vi "Decoder.vi"(8 "Joystick Data":string, 9 "Button Data":string, 10 "Conf":T3) -> (1 "Controller 2 State":T1={"Left X"=0, "Left Y"=0, "Right X"=0, "Right Y"=0, "Button Encoding 9-12"=0, "Button Encoding 1-8"=0, "POV"=-1} {"POV" items=["None"=-1, "POV Up"=0, "POV Up Right"=1, "POV Right"=2, "POV Down Right"=3, "POV Down"=4, "POV Down Left"=5, "POV Left"=6, "POV Up Left"=7]}, 2 "Controller 1 State":T1={"Left X"=0, "Left Y"=0, "Right X"=0, "Right Y"=0, "Button Encoding 9-12"=0, "Button Encoding 1-8"=0, "POV"=-1} {"POV" items=["None"=-1, "POV Up"=0, "POV Up Right"=1, "POV Right"=2, "POV Down Right"=3, "POV Down"=4, "POV Down Left"=5, "POV Left"=6, "POV Up Left"=7]})   [LabVIEW 2010, in "Packet Recorder.lvlib"]
uses:
  Packet Recorder.lvlib
  <vilib>/FTC/FTC ControllerState.ctl
  <vilib>/FTC/FTC POVState.ctl
  Components/Components.llb/Integer to Boolean Array_U32.vi
  Components/Components.lvlib
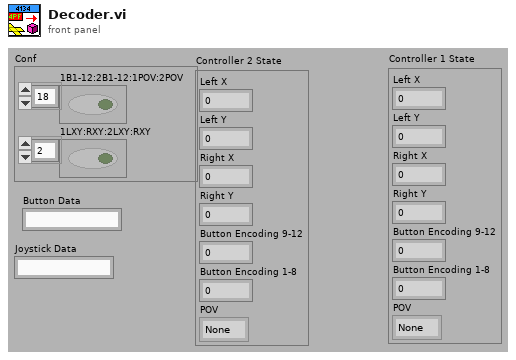
[diagram p1: front panel]
types:
  T1 = typedef "FTC ControllerState.ctl" = cluster{"Left X":i8, "Left Y":i8, "Right X":i8, "Right Y":i8, "Button Encoding 9-12":u8, "Button Encoding 1-8":u8, "POV":T2}
  T2 = typedef "FTC POVState.ctl" = i8
  T3 = cluster{"1B1-12:2B1-12:1POV:2POV":bool[], "1LXY:RXY:2LXY:RXY":bool[]}
  T4 = enum16{"big-endian, network order", "native, host order", "little-endian"}
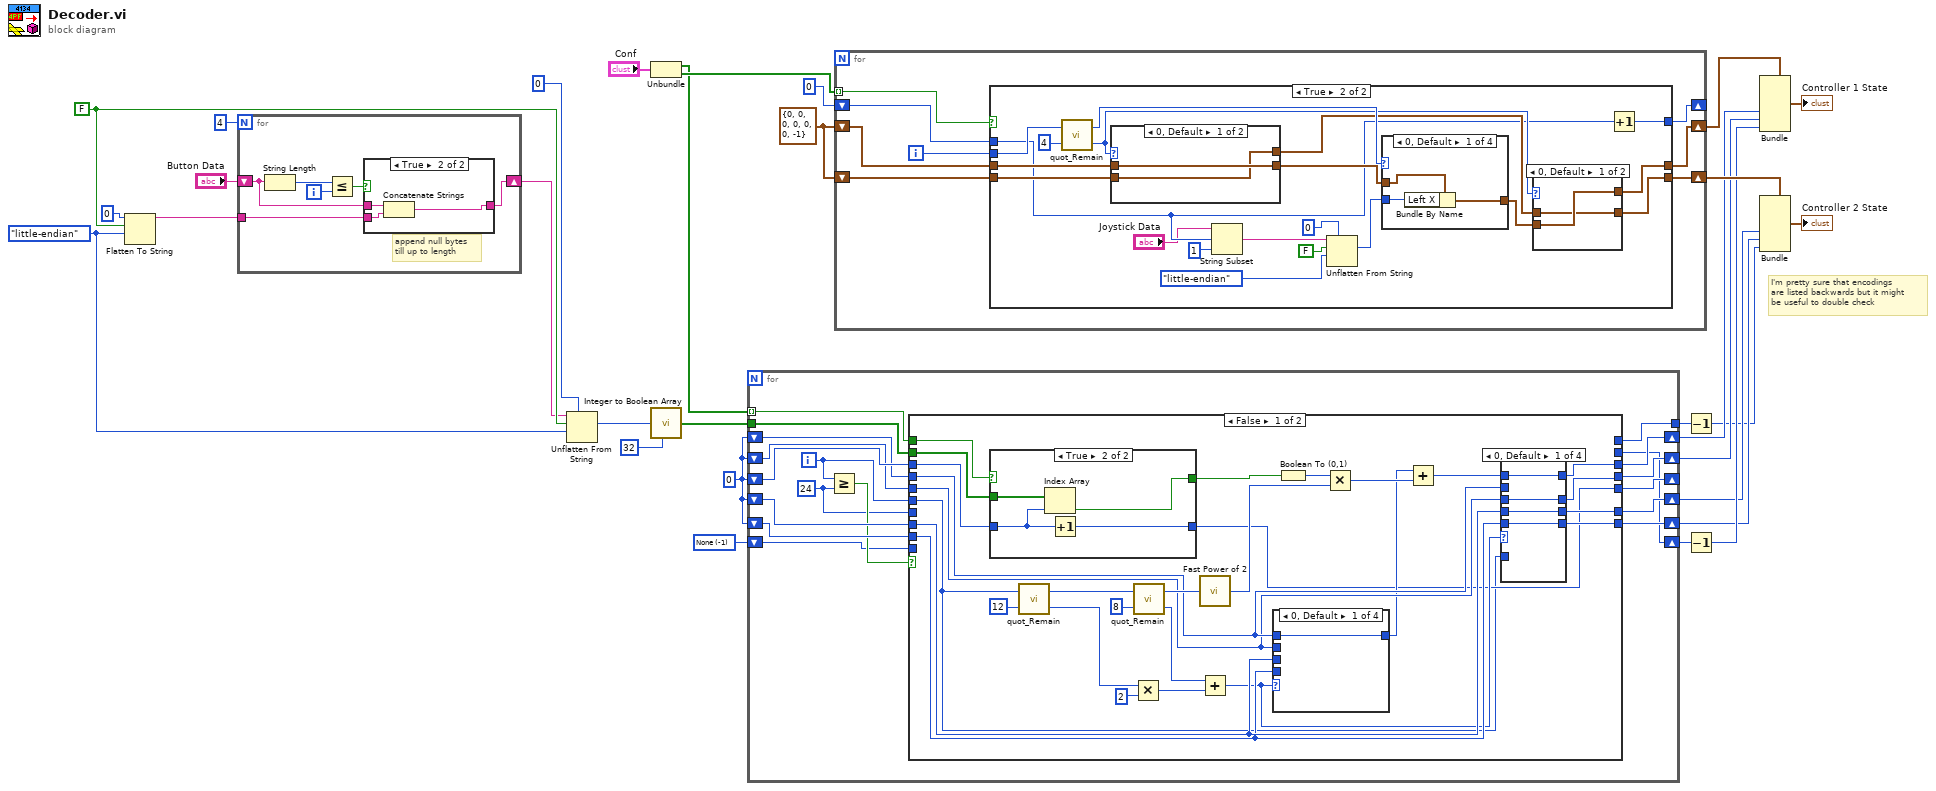
[diagram p0: block diagram]
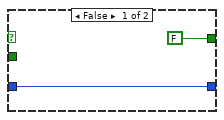
[diagram p9: hidden frame]
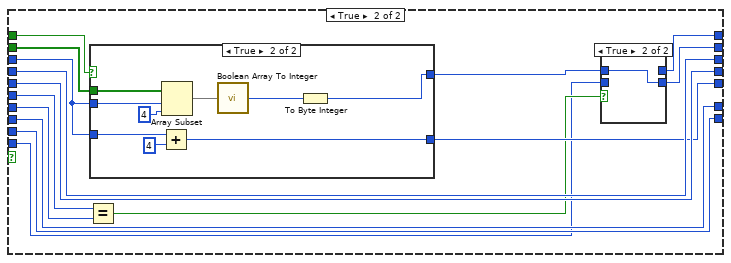
[diagram p10: hidden frame]
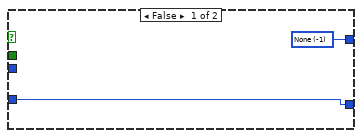
[diagram p12: hidden frame]
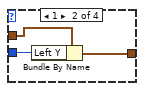
[diagram p16: hidden frame]
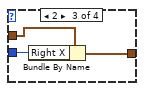
[diagram p17: hidden frame]
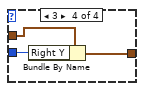
[diagram p18: hidden frame]
diagram:
  w11 = T2 -1 items=["None"=-1, "POV Up"=0, "POV Up Right"=1, "POV Right"=2, "POV Down Right"=3, "POV Down"=4, "POV Down Left"=5, "POV Left"=6, "POV Up Left"=7] ("POV")
  w17 = u8 0 ("index")
  w15 = FALSE ("data includes array or string size? (T)")
  w14 = T4."little-endian" ("byte order (0:big-endian, network order)")
  w28 = T1 {"Left X"=0, "Left Y"=0, "Right X"=0, "Right Y"=0, "Button Encoding 9-12"=0, "Button Encoding 1-8"=0, "POV"=-1} ("Controller 2 State")
  # "I'm pretty sure that encodings \nare listed backwards but it might\nbe useful to double check"
  n1 = Flatten To String(anything=u8 0, prepend array or string size? (T)=w15, byte order (0:big-endian, network order)=w14) -> (data string=w6:string)  [unwired: 1 in, 2 out]
  n2 = for {
    N: 4 -> [_]
    tunnel: w6 -> [w36]
    shift-right: [w35] -> w5
    shift-left: "Button Data" -> [w33]
    i -> [w32]
    # "append null bytes\ntill up to length"
    n3 = String Length(string=w33) -> (length=w34:i32)
    n4 = Less Or Equal?(x=w34, y=w32) -> (x <= y?=w31:bool)
    n5 = case shown="True" w31 {
      tunnel: w33 -> [w37 w40]
      tunnel: w36 -> [_ w39]
      tunnel: [w37 w38] -> w35
      frame False {
      }
      frame True {
        n6 = Concatenate Strings(w40, w39) -> (w38:string)
      }
    }
  }
  n7 = Unflatten From String(type=u32 0, binary string=w5, data includes array or string size? (T)=w15, byte order (0:big-endian, network order)=w14) -> (value=w9:u32)  [unwired: 1 in, 2 out]
  n8 = Unbundle("Conf") -> ("1B1-12:2B1-12:1POV:2POV"=w26:bool[], "1LXY:RXY:2LXY:RXY"=w27:bool[])
  n9 = call-poly "Integer to Boolean Array.vi"("number"=w9, "minimum"=u32 32) -> ("Boolean array"=w4:bool[])  [unwired: 5 in]
  n10 = for {
    tunnel: w26 -> [w58] mode=indexing
    tunnel: w4 -> [w57]
    shift-right: [w55] -> _
    shift-left: w17 -> [w56]
    shift-right: [w54] -> w19
    shift-left: w17 -> [w50]
    shift-right: [w51] -> w2
    shift-left: w17 -> [w47]
    shift-right: [w52] -> w3
    shift-left: w17 -> [w48]
    shift-right: [w53] -> w18
    shift-left: w17 -> [w49]
    shift-right: [w43] -> w13
    shift-left: w11 -> [w42]
    tunnel: [w41] -> w12
    i -> [w45]
    w44 = 24 ("y")
    n11 = Greater Or Equal?(x=w45, y=w44) -> (x >= y?=w46:bool)
    n12 = case shown="False" w46 {
      tunnel: w58 -> [w60 w121]
      tunnel: w57 -> [w86 w120]
      tunnel: w56 -> [w85 w119]
      tunnel: [w62 w123] -> w55
      tunnel: w45 -> [w59 w113]
      tunnel: [w73 w127] -> w54
      tunnel: [w72 w126] -> w53
      tunnel: [w71 w124] -> w52
      tunnel: [w70 w125] -> w51
      tunnel: w50 -> [w69 w127]
      tunnel: w49 -> [w68 w126]
      tunnel: w48 -> [w67 w124]
      tunnel: w47 -> [w66 w125]
      tunnel: w44 -> [_ w122]
      tunnel: [_ w116] -> w43
      tunnel: w42 -> [_ w115]
      tunnel: [_ w114] -> w41
      frame False {
        n13 = case shown="True" w60 {
          tunnel: w86 -> [_ w112]
          tunnel: w85 -> [w108 w111]
          tunnel: [w108 w110] -> w62
          tunnel: [FALSE w109] -> w61
          frame False {
          }
          frame True {
            n14 = Index Array(array=w112, index=w111) -> (element=w109:bool)
            n15 = Increment(x=w111) -> (x+1=w110:u8)
          }
        }
        n16 = call <vilib>:"quot_Remain.vi"("y"=12, "x"=w59) -> ("floor(x/y)"=w78:i32, "x-y*floor(x/y)"=w83:i32)
        n17 = Multiply(x=w78, y=2) -> (x*y=w76:i32)
        n18 = call <vilib>:"quot_Remain.vi"("y"=8, "x"=w83) -> ("floor(x/y)"=w75:i32, "x-y*floor(x/y)"=w81:i32)
        n19 = call "Fast Power of 2.vi"("power"=w81) -> ("result"=w80:u32)
        n20 = Add(x=w75, y=w76) -> (x+y=w63:i32)
        n21 = case shown="0, Default" w63 {
          tunnel: w69 -> [w87 _ _ _]
          tunnel: w68 -> [_ w88 _ _]
          tunnel: w67 -> [_ _ w89 _]
          tunnel: w66 -> [_ _ _ w90]
          tunnel: [w87 w88 w89 w90] -> w65
          frame 0, Default {
          }
          frame 1 {
          }
          frame 2 {
          }
          frame 3 {
          }
        }
        n22 = Boolean To (0,1)(Boolean=w61) -> (0, 1=w64:i16)
        n23 = Multiply(x=w64, y=w80) -> (x*y=w79:u32)
        n24 = Add(x=w65, y=w79) -> (x+y=w74:u32)
        n25 = case shown="0, Default" w63 {
          tunnel: w74 -> [w91 w98 w102 w106]
          tunnel: [w91 w97 w101 w105] -> w73
          tunnel: [w92 w98 w100 w104] -> w72
          tunnel: [w93 w96 w102 w103] -> w71
          tunnel: [w94 w95 w99 w106] -> w70
          tunnel: w66 -> [w94 w95 w99 _]
          tunnel: w67 -> [w93 w96 _ w103]
          tunnel: w68 -> [w92 _ w100 w104]
          tunnel: w69 -> [_ w97 w101 w105]
          tunnel: w59 -> [_ _ _ _]
          frame 0, Default {
          }
          frame 1 {
          }
          frame 2 {
          }
          frame 3 {
          }
        }
      }
      frame True {
        n26 = Equal?(x=w113, y=w122) -> (x = y?=w117:bool)
        n27 = case shown="True" w121 {
          tunnel: w119 -> [w131 w141]
          tunnel: [w131 w140] -> w123
          tunnel: w120 -> [_ w136]
          tunnel: w119 -> [_ w135]
          tunnel: [w132 w133] -> w118
          frame False {
            w132 = T2 -1 items=["None"=-1, "POV Up"=0, "POV Up Right"=1, "POV Right"=2, "POV Down Right"=3, "POV Down"=4, "POV Down Left"=5, "POV Left"=6, "POV Up Left"=7] ("POV")
          }
          frame True {
            n28 = Add(x=w141, y=u8 4) -> (x+y=w140:u8)
            n29 = Array Subset(array=w136, index=w135, length=4) -> (w137:bool[])
            n30 = call "Boolean Array To Integer.vi"("Boolean array"=w137) -> ("number"=w134:u32)  [unwired: 4 in]
            n31 = To Byte Integer(number=w134) -> (8bit integer=w133:i8)
          }
        }
        n32 = case shown="True" w117 {
          tunnel: w118 -> [w128 w130]
          tunnel: [w129 w130] -> w116
          tunnel: w115 -> [w129 _]
          tunnel: [w128 _] -> w114
          frame False {
          }
          frame True {
          }
        }
      }
    }
  }
  n33 = for {
    shift-right: [w146] -> w23
    shift-left: w28 -> [w148]
    shift-right: [w142] -> _
    shift-left: u8 0 -> [w143]
    shift-right: [w145] -> w22
    shift-left: w28 -> [w147]
    tunnel: w27 -> [w144] mode=indexing
    i -> [w149]
    n34 = case shown="True" w144 {
      tunnel: w149 -> [_ w171]
      tunnel: w148 -> [w152 w169]
      tunnel: w147 -> [w151 w168]
      tunnel: [w152 w164] -> w146
      tunnel: [w151 w163] -> w145
      tunnel: w143 -> [w150 w159]
      tunnel: [w150 w161] -> w142
      frame False {
      }
      frame True {
        n35 = call <vilib>:"quot_Remain.vi"("y"=4, "x"=w171) -> ("floor(x/y)"=w167:i32, "x-y*floor(x/y)"=w170:i32)
        n36 = case shown="0, Default" w167 {
          tunnel: w169 -> [w178 w179]
          tunnel: w168 -> [w177 w180]
          tunnel: [w178 w180] -> w166
          tunnel: [w177 w179] -> w162
          frame 0, Default {
          }
          frame 1 {
          }
        }
        n37 = String Subset(string="Joystick Data", offset (0)=w159, length (rest)=1 ("length (rest)")) -> (substring=w156:string)
        n38 = Unflatten From String(type=i8 0, binary string=w156, data includes array or string size? (T)=FALSE, byte order (0:big-endian, network order)=T4."little-endian") -> (value=w153:i8)  [unwired: 1 in, 2 out]
        n39 = case shown="0, Default" w170 {
          tunnel: w166 -> [w183 w186 w188 w192]
          tunnel: [w182 w185 w189 w191] -> w165
          tunnel: w153 -> [w181 w184 w187 w190]
          frame 0, Default {
            n40 = Bundle By Name(cluster=w183, "Left X"=w181) -> (w182:T1)
          }
          frame 1 {
            n41 = Bundle By Name(cluster=w186, "Left Y"=w184) -> (w185:T1)
          }
          frame 2 {
            n42 = Bundle By Name(cluster=w188, "Right X"=w187) -> (w189:T1)
          }
          frame 3 {
            n43 = Bundle By Name(cluster=w192, "Right Y"=w190) -> (w191:T1)
          }
        }
        n44 = case shown="0, Default" w167 {
          tunnel: w165 -> [w174 w176]
          tunnel: [w174 w175] -> w164
          tunnel: [w173 w176] -> w163
          tunnel: w162 -> [w173 w175]
          frame 0, Default {
          }
          frame 1 {
          }
        }
        n45 = Increment(x=w159) -> (x+1=w161:u8)
      }
    }
  }
  n46 = Decrement(x=w12) -> (x-1=w1:T2)
  n47 = Decrement(x=w13) -> (x-1=w10:T2)
  n48 = Bundle(cluster=w23, "Button Encoding 9-12"=w19, "Button Encoding 1-8"=w18, "POV"=w10) -> (→"Controller 1 State":T1)  [unwired: 4 in]
  n49 = Bundle(cluster=w22, "Button Encoding 9-12"=w3, "Button Encoding 1-8"=w2, "POV"=w1) -> (→"Controller 2 State":T1)  [unwired: 4 in]
